vi "example_GRecord.vi"() -> ()   [LabVIEW 2021]
uses:
  <vilib>/Galil/resources/gclib/gclib.lvlib
panel:
  out "TIME":u16
  in  "IP Address":string="192.168.1.77 --subscribe DR"
  out "Controller ID":string
  out "error out":errorcluster
  in  "stop":bool
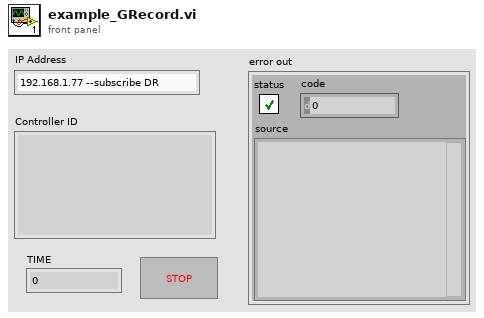
[diagram p1: front panel]
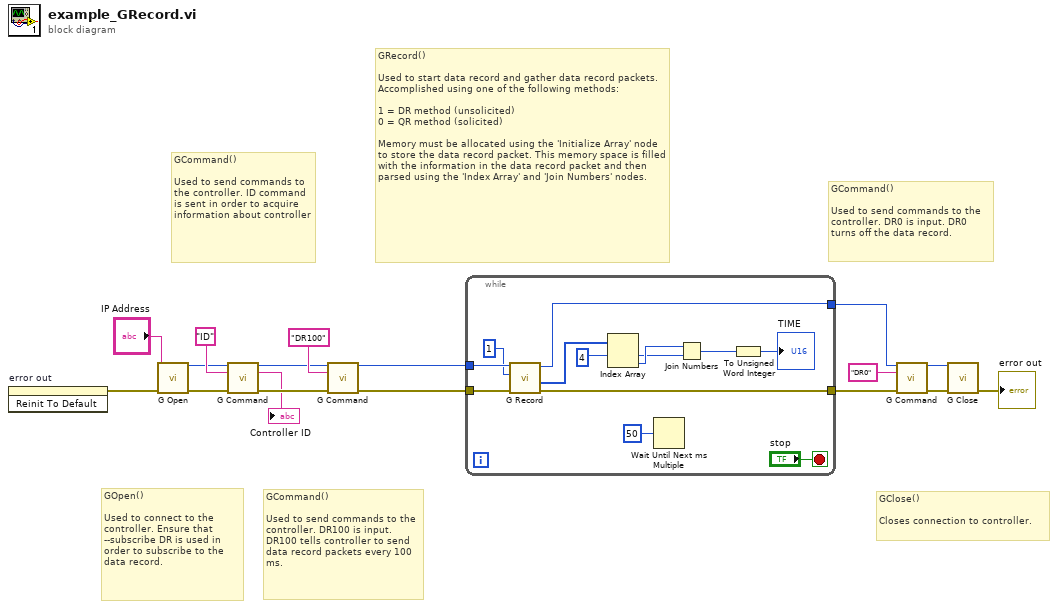
[diagram p0: block diagram]
diagram:
  # "GRecord()\n\nUsed to start data record and gather data record packets. Accomplished using one of the following methods:\n\n1 = DR method (unsolicited)\n0 = QR method (solicited)\n\nMemory must be allocated using the 'Initialize Array' node to store the data record packet. This memory space is filled with the information in the data record packet and then parsed using the 'Index Array' and 'Join Numbers' nodes."
  # "GClose()\n\nCloses connection to controller."
  # "GCommand()\n\nUsed to send commands to the controller. DR0 is input. DR0 turns off the data record."
  # "GCommand()\n\nUsed to send commands to the controller. DR100 is input. DR100 tells controller to send data record packets every 100 ms."
  # "GCommand()\n\nUsed to send commands to the controller. ID command is sent in order to acquire information about controller"
  # "GOpen()\n\nUsed to connect to the controller. Ensure that \n--subscribe DR is used in order to subscribe to the data record."
  n1 = invoke on="error out" class="Clust (strict)" method="Reinit To Default"() -> (error out=w3:errorcluster)  [unwired: 3 in, 2 out]
  n2 = call <vilib>:"G Open.vi"("error in (no error)"=w3, "address"="IP Address") -> ("error out"=w2:errorcluster, "g out"=w1:u64)  [unwired: 7 in]
  n3 = call <vilib>:"G Command.vi"("g"=w1, "command"="ID" ("buffer"), "error in (no error)"=w2) -> ("g out"=w10:u64, "buffer out"=→"Controller ID":string, "error out"=w9:errorcluster)  [unwired: 10 in]
  n4 = call <vilib>:"G Command.vi"("g"=w10, "command"="DR100", "error in (no error)"=w9) -> ("g out"=w6:u64, "error out"=w5:errorcluster)  [unwired: 10 in, 1 out]
  n5 = while {
    tunnel: [w20] -> w15
    tunnel: [w22] -> w13
    tunnel: w6 -> [w25]
    tunnel: w5 -> [w23]
    stop <- "stop" stop-if-true
    n6 = call <vilib>:"G Record.vi"("error in (no error)"=w23, "method"=1, "g"=w25) -> ("error out"=w20:errorcluster, "record out"=w21:u8[], "g out"=w22:u64)  [unwired: 6 in]
    n7 = Index Array "Index Array"(array=w21, index #1=4 ("index")) -> (element #1=w27:u8, element #2=w28:u8)  [unwired: 1 in]
    n8 = Wait Until Next ms Multiple(millisecond multiple=u32 50) -> ()  [unwired: 1 out]
    n9 = Join Numbers(hi=w28, lo=w27) -> ((hi.lo)=w19:u16)
    n10 = To Unsigned Word Integer(number=w19) -> (unsigned 16bit integer=→"TIME":u16)
  }
  n11 = call <vilib>:"G Command.vi"("g"=w13, "command"="DR0", "error in (no error)"=w15) -> ("g out"=w12:u64, "error out"=w14:errorcluster)  [unwired: 10 in, 1 out]
  n12 = call <vilib>:"G Close.vi"("error in (no error)"=w14, "g"=w12) -> ("error out"=→"error out":errorcluster)  [unwired: 9 in]
